vi "一体站流程质控自动启动.vi"(6 "CODMn量程切换":enum32{"H", "L", "AUTO"}(ring)=enum."AUTO", 8 "总磷量程切换":enum32{"H", "L", "AUTO"}(ring)=enum."AUTO", 9 "总氮量程切换":enum32{"H", "L", "AUTO"}(ring)=enum."AUTO", 10 "氨氮量程切换":enum32{"H", "L", "AUTO"}(ring)=enum."AUTO", 11 "参数":T1={"是否启用仪器"=FALSE, "CODMn"={"启动测量模式"={"测量模式"=enum."水样测量"}, "确定按钮"=TRUE}, "启动模块"={"氨氮"=FALSE, "总磷"=FALSE, "总氮"=FALSE, "CODMn"=FALSE, "CODCr"=FALSE}, "常规启动"=FALSE, "直接启动"=FALSE}) -> ()   [LabVIEW 2016, in "质控单元.lvlib"]
panel:
  out "枚举 2":enum16{"初始化", "采配水启动", "等待", "配水", "排水", "结束"}(ring)
  out "枚举":enum16{"初始化", "采配水启动", "等待", "配水", "排水", "结束"}(ring)
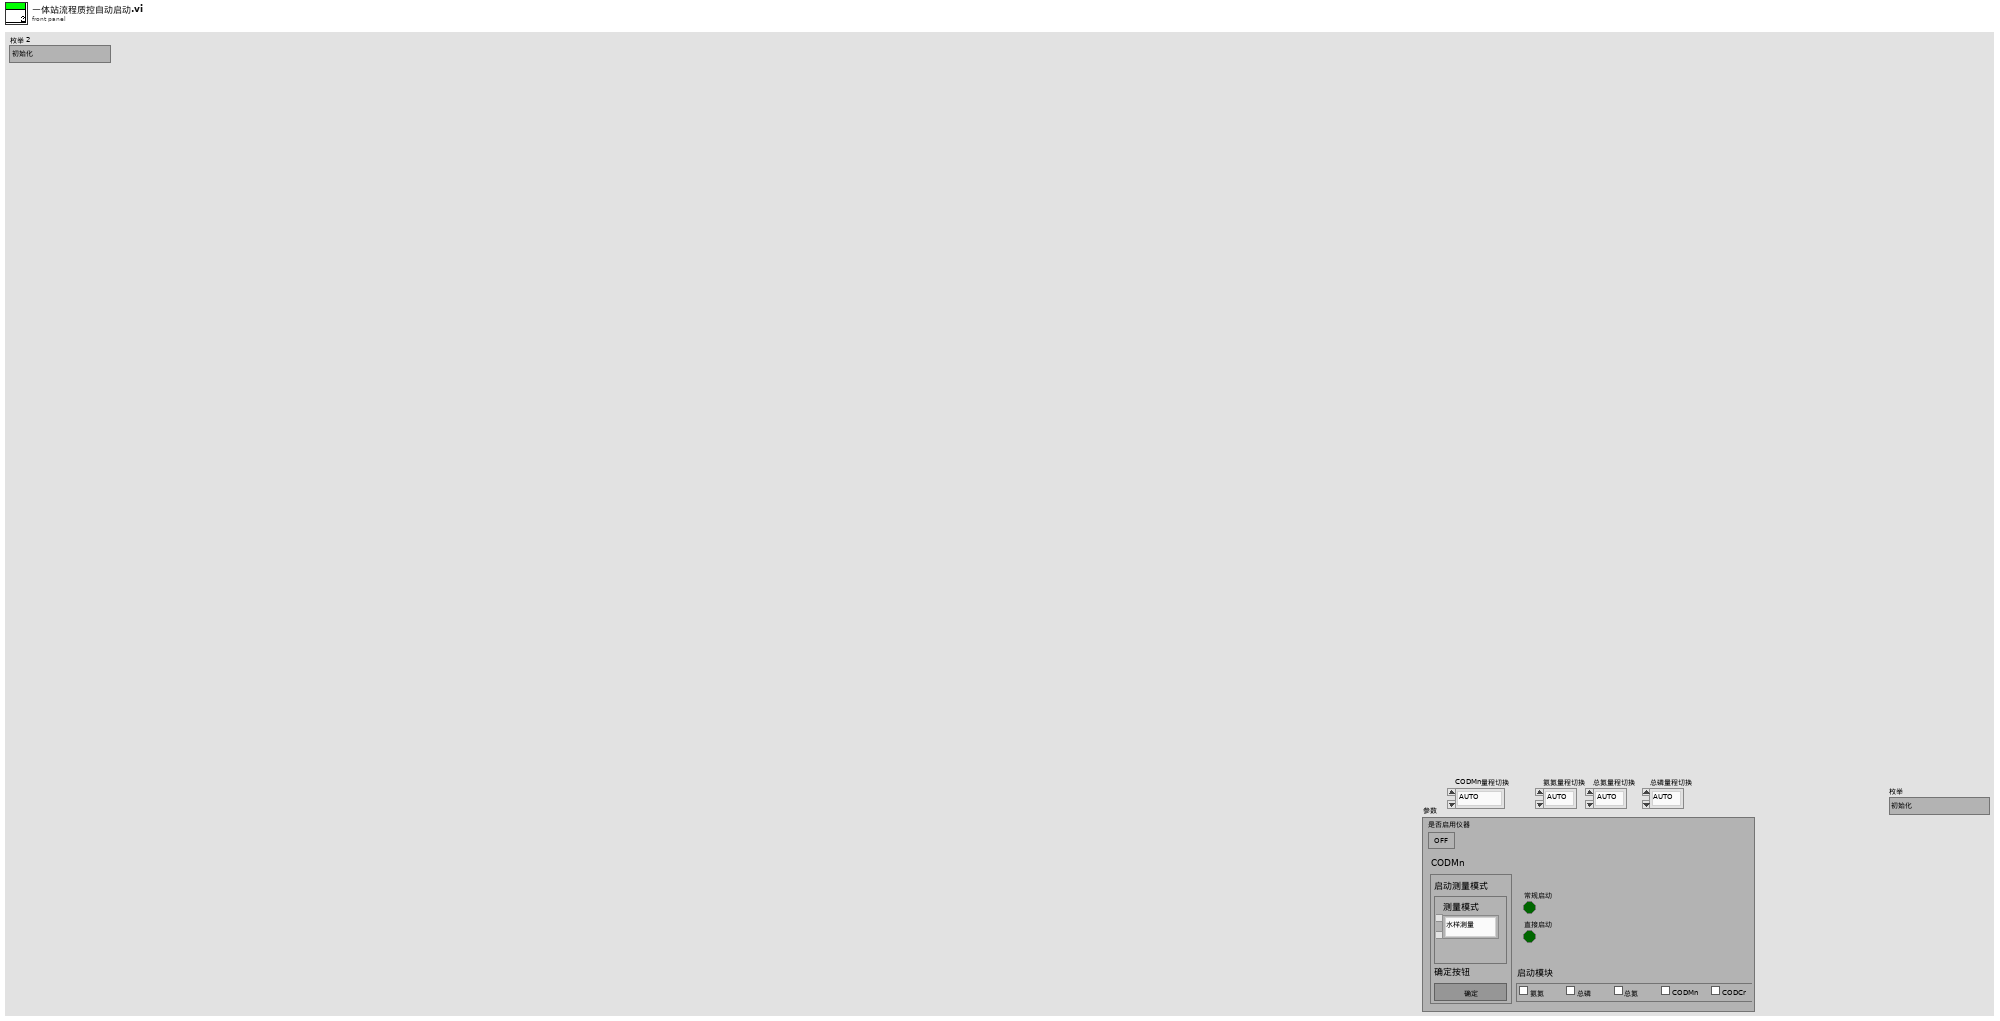
[diagram p1: front panel]
types:
  T1 = cluster{"是否启用仪器":bool, "CODMn":cluster{"启动测量模式":cluster{"测量模式":enum16{"水样测量", "标样核查", "加标回收", "平行样", "校零", "校标"}}, "确定按钮":bool}, "启动模块":cluster{"氨氮":bool, "总磷":bool, "总氮":bool, "CODMn":bool, "CODCr":bool}, "常规启动":bool, "直接启动":bool}
  T2 = cluster{"命令":string, cluster{"starting address":u16, "holding register value":u16}}
  T3 = cluster{"R0":i16, "R1":i16, "R2":i16, "R3":i16, "R4":i16, "R5":i16, "R6":i16, "R7":i16, "R8":i16, "R9":i16, "R10":i16, "R11":i16, "R12":i16, "R13":i16, "R14":i16, "R15":i16, "R16":i16, "R17":i16, "R18":i16, "R19":i16, "R20":i16, "R21":i16, "R22":i16, "R23":i16, "R24":i16, "R25":i16, "R26":i16, "R27":i16, "R28":i16, "R29":i16, "R30":i16, "R31":i16, "R32":i16, "R33":i16, "R34":i16, "R35":i16, "R36":i16, "R37":i16, "R38":i16, "R39":i16, "R40":i16, "R41":i16, "R42":i16, "R43":i16, "R44":i16, "R45":i16, "R46":i16, "R47":i16, "R48":i16, "R49":i16, "R50":i16, "R51":i16, "R52":i16, "R53":i16, "R54":i16, "R55":i16, "R56":i16}
  T4 = enum32{"Bad", "Idle", "Run top level", "Running"}
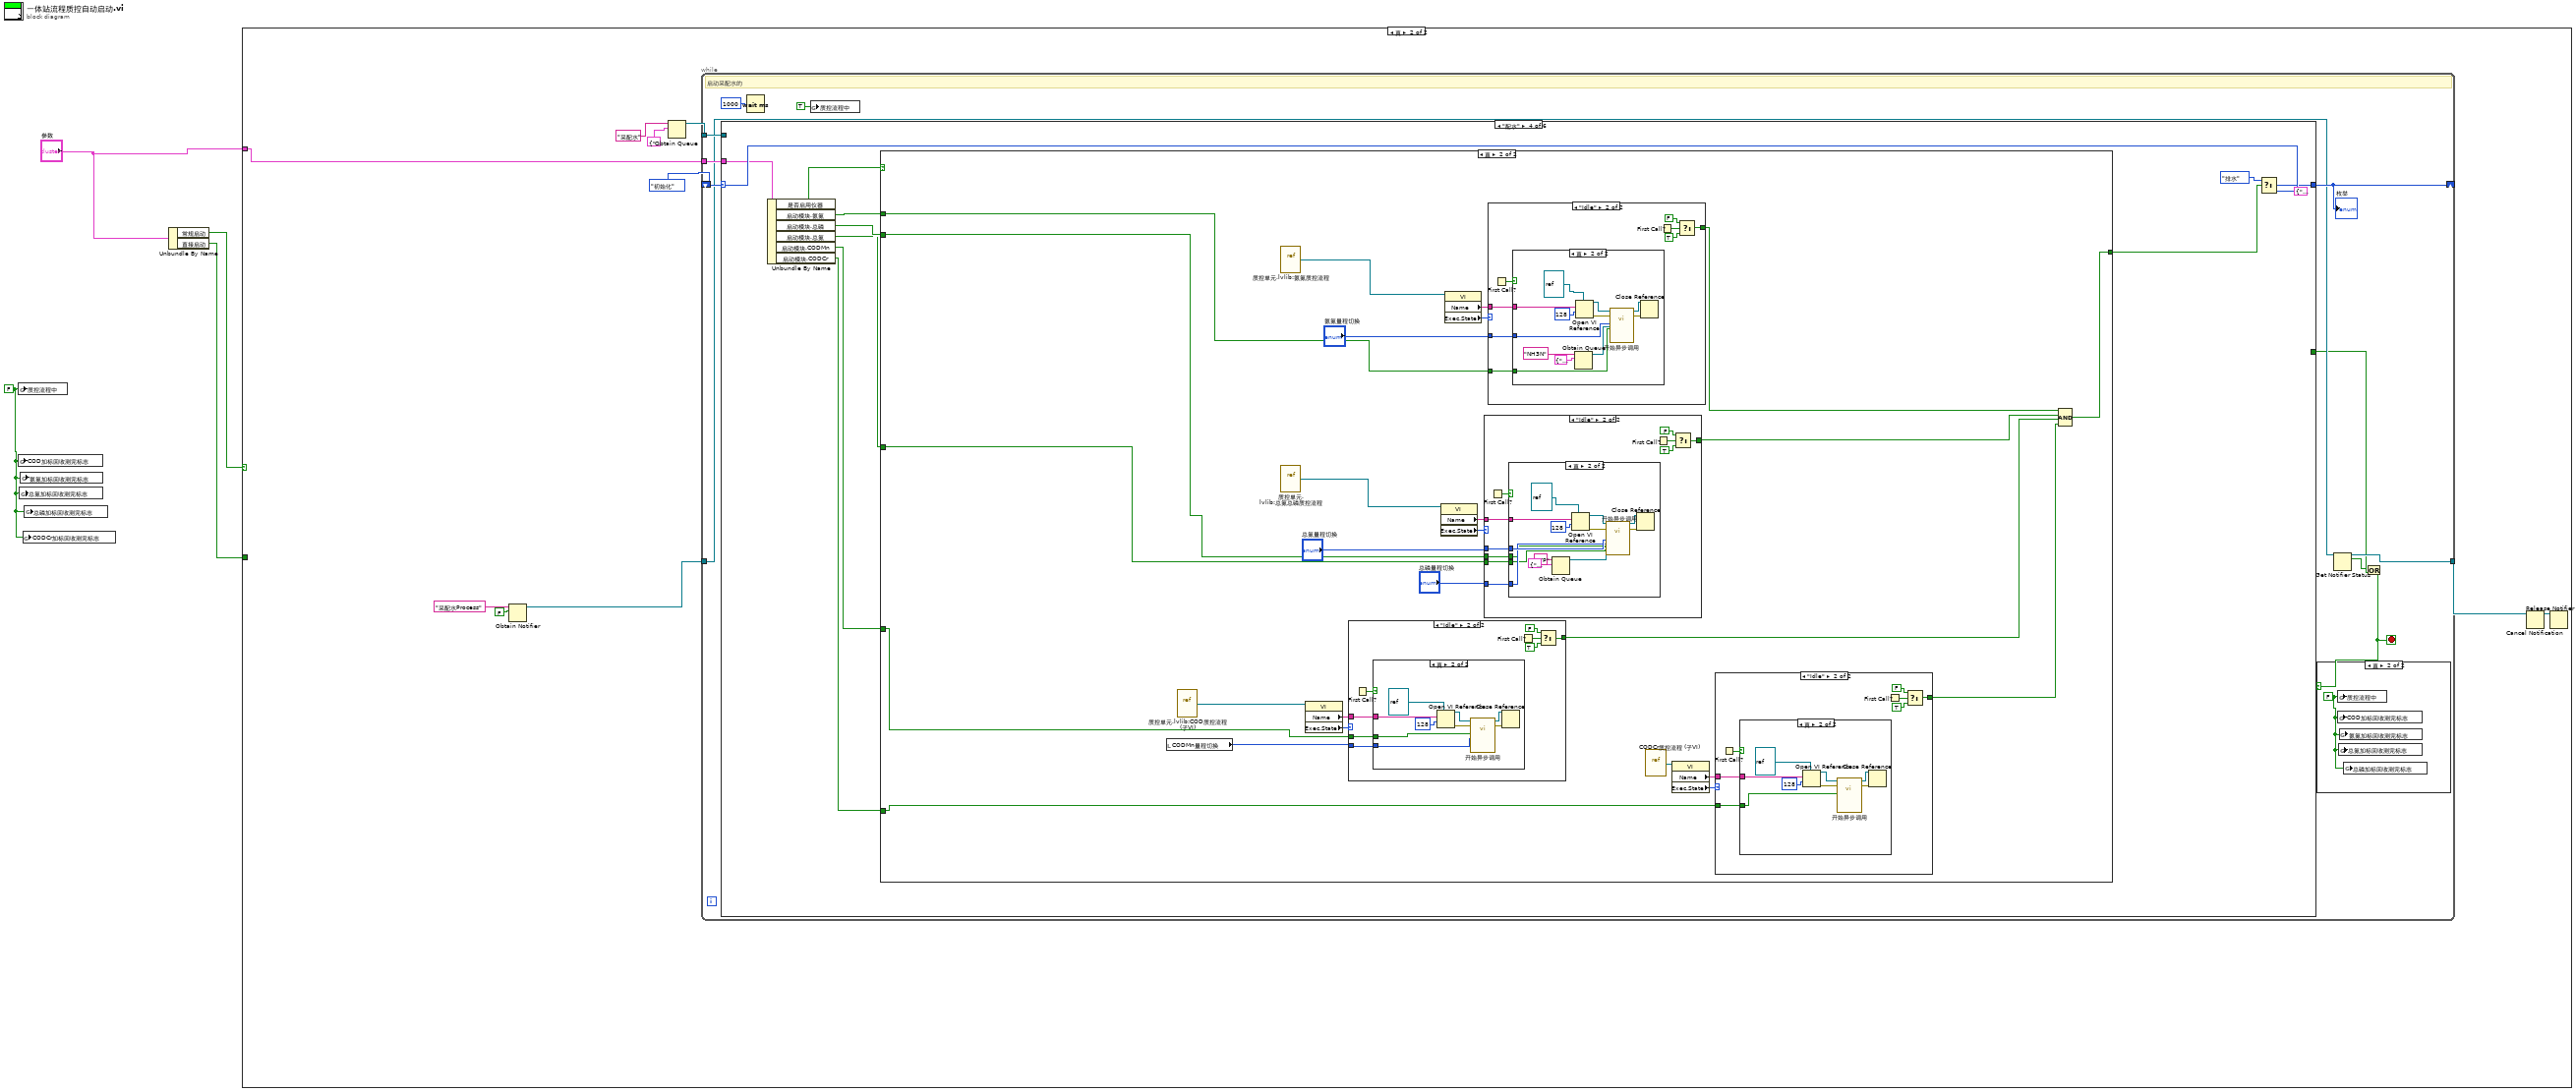
[diagram p0: block diagram]
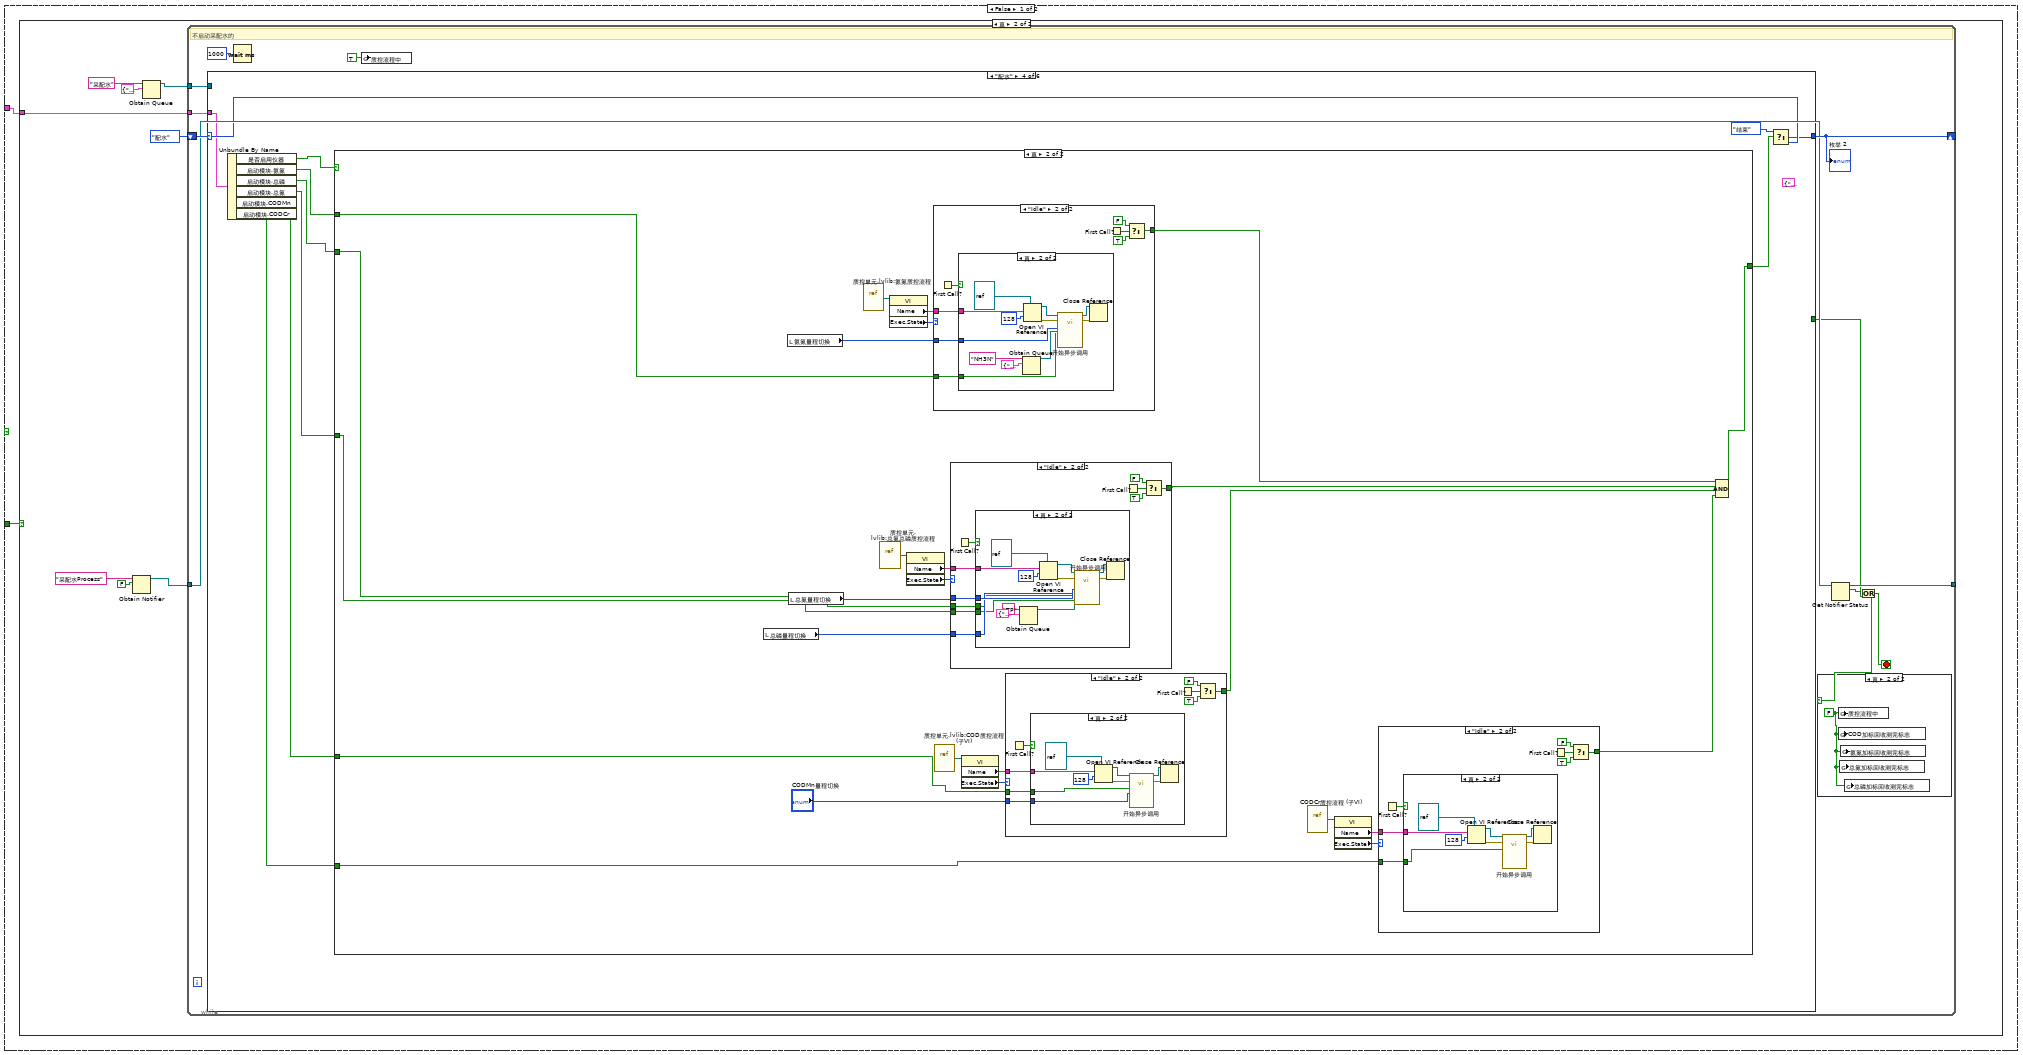
[diagram p2: hidden frame]
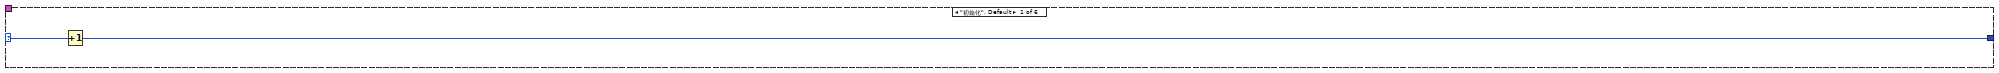
[diagram p5: hidden frame]
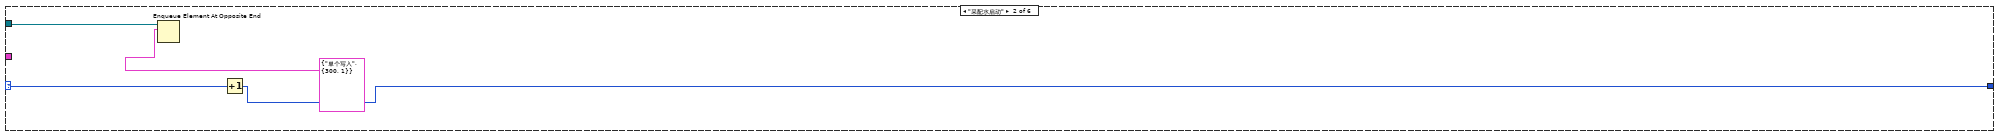
[diagram p6: hidden frame]
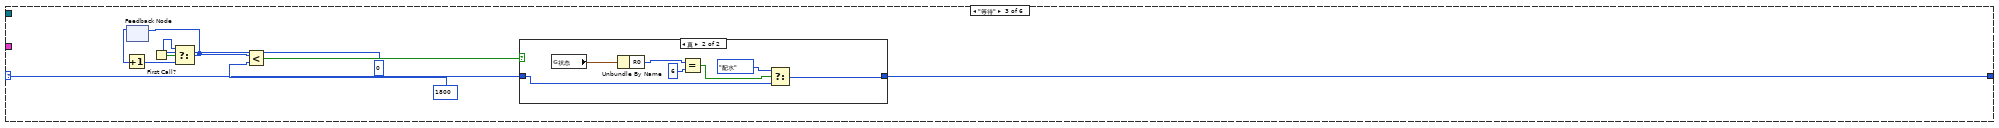
[diagram p7: hidden frame]
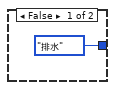
[diagram p8: hidden frame]
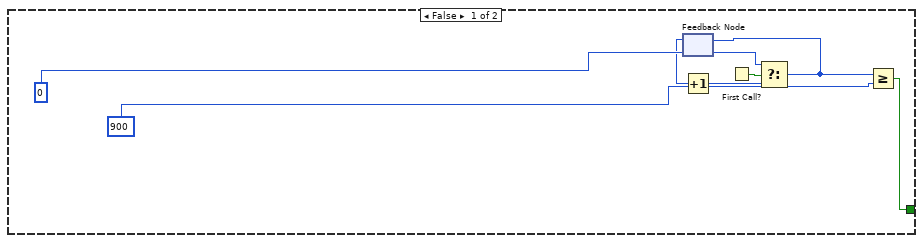
[diagram p9: hidden frame]
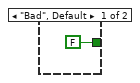
[diagram p10: hidden frame]
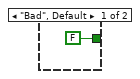
[diagram p12: hidden frame]
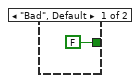
[diagram p14: hidden frame]
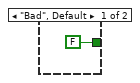
[diagram p16: hidden frame]
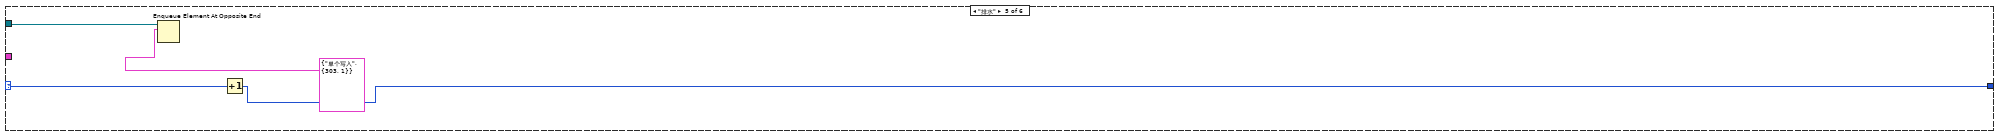
[diagram p18: hidden frame]
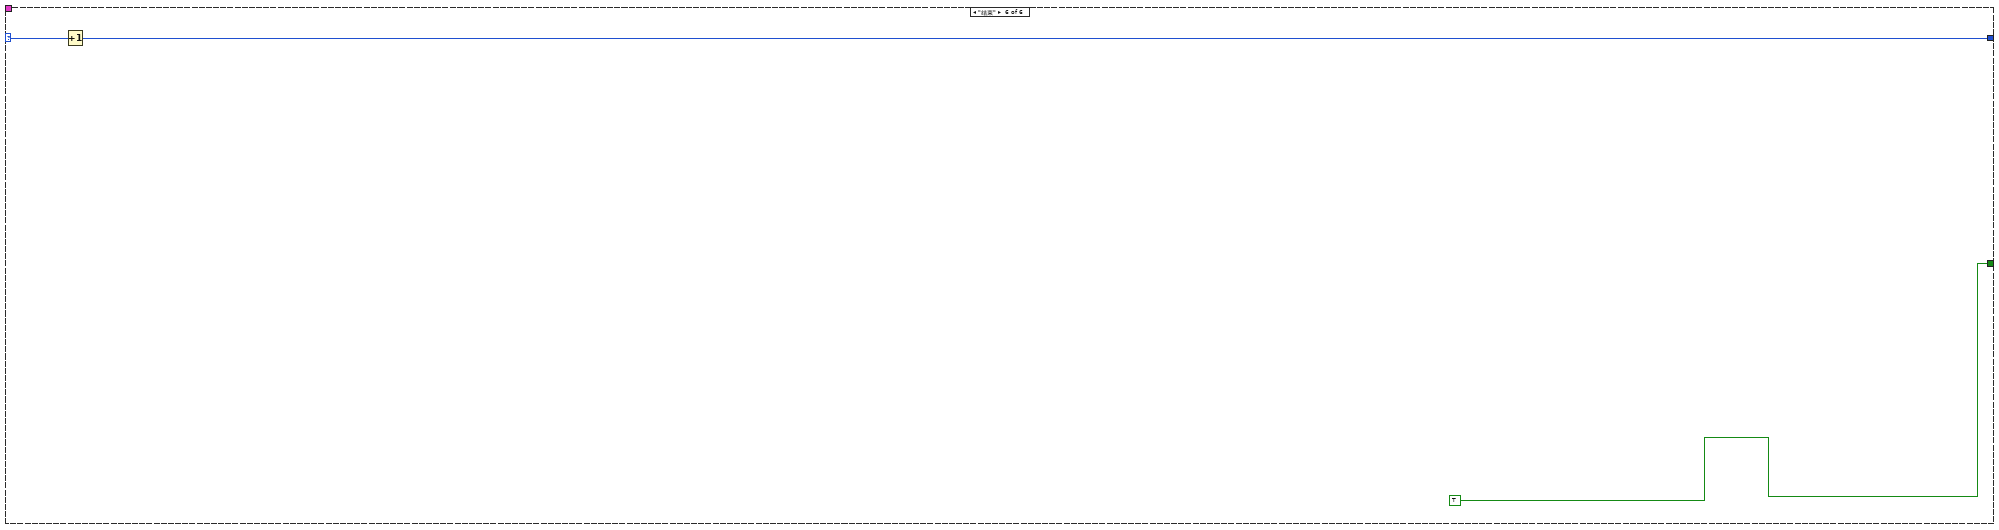
[diagram p19: hidden frame]
diagram:
  w1 = FALSE ("质控流程中")
  n1 = global write "质控测完标志全局 1.vi" "质控流程中"(w1) -> ()
  n2 = global write "质控测完标志全局 1.vi" "COD加标回收测完标志"(w1) -> ()
  n3 = global write "质控测完标志全局 1.vi" "总氮加标回收测完标志"(w1) -> ()
  n4 = global write "质控测完标志全局 1.vi" "氨氮加标回收测完标志"(w1) -> ()
  n5 = global write "质控测完标志全局 1.vi" "CODCr加标回收测完标志"(w1) -> ()
  n6 = global write "质控测完标志全局 1.vi" "总磷加标回收测完标志"(w1) -> ()
  n7 = Unbundle By Name("参数") -> ("常规启动"=w3:bool, "直接启动"=w2:bool)
  n8 = case shown="真" w3 {
    tunnel: "参数" -> [w5 w181]
    tunnel: w2 -> [w6 _]
    frame False {
      n9 = case shown="真" w6 {
        tunnel: w5 -> [_ w13]
        frame False {
        }
        frame True {
          n10 = Obtain Notifier(name (unnamed)="采配水Process" ("名称（未命名）"), notification data type=FALSE) -> (notifier out=w7:refnum<notifier>)  [unwired: 2 in, 2 out]
          n11 = Obtain Queue(name (unnamed)="采配水" ("名称（未命名）"), element data type=cluster{"命令":string, "数据":variant} {"命令"="", "数据"=variant}) -> (queue out=w10:refnum<queue>)  [unwired: 3 in, 2 out]
          n12 = while {
            tunnel: w10 -> [w25]
            shift-right: [w23] -> _
            shift-left: enum16{"初始化", "采配水启动", "等待", "配水", "排水", "结束"}."配水" ("枚举") -> [w24]
            tunnel: w13 -> [w21]
            tunnel: w7 -> [w20]
            tunnel: [w19] -> _
            stop <- w16 stop-if-true
            # "不启动采配水的"
            n13 = case shown="\"配水\"" w24 {
              selector: w24 -> [w28 w30 w39 w59 w175 w180]
              tunnel: w25 -> [_ w31 _ _ w176 _]
              tunnel: [w27 w29 w38 w58 w174 w179] -> w23
              tunnel: [_ _ _ _ _ TRUE] -> w18
              tunnel: w21 -> [_ _ _ w55 _ _]
              frame "初始化", Default {
                n14 = Increment(x=w28) -> (x+1=w27:enum16{"初始化", "采配水启动", "等待", "配水", "排水", "结束"})
              }
              frame "采配水启动" {
                n15 = Enqueue Element At Opposite End(queue=w31, element=T2 {"命令"="单个写入", {"starting address"=300, "holding register value"=1}} ("元素")) -> ()  [unwired: 2 in, 3 out]
                n16 = Increment(x=w30) -> (x+1=w29:enum16{"初始化", "采配水启动", "等待", "配水", "排水", "结束"})
              }
              frame "等待" {
                n17 = feedback #1() -> (w35:i32)  [unwired: 1 in]
                n18 = Increment(x=w35) -> (x+1=w34:i32)
                n19 = First Call?() -> (First Call?: T/F=w36:bool)
                n20 = Select(t=0, s=w36, f=w34) -> (s? t:f=w33:i32)
                n21 = feedback-in #1(w33) -> ()
                n22 = Less?(x=w33, y=1800) -> (x < y?=w40:bool)
                n23 = case shown="真" w40 {
                  tunnel: w39 -> [_ w45]
                  tunnel: [enum16{"初始化", "采配水启动", "等待", "配水", "排水", "结束"}."排水" ("枚举") w44] -> w38
                  frame False {
                  }
                  frame True {
                    n24 = global read "与采配水交互全局.vi" "状态"() -> (w43:T3)
                    n25 = Unbundle By Name(w43) -> ("R0"=w49:i16)
                    n26 = Equal?(x=w49, y=i16 6) -> (x = y?=w47:bool)
                    n27 = Select(t=enum16{"初始化", "采配水启动", "等待", "配水", "排水", "结束"}."配水" ("枚举"), s=w47, f=w45) -> (s? t:f=w44:enum16{"初始化", "采配水启动", "等待", "配水", "排水", "结束"})
                  }
                }
              }
              frame "配水" {
                (unwired) cluster{"命令":string, "data":variant} {"命令"="启动", "data"=variant(cluster{"站号":u16, "控制命令输出":u16[]} {"站号"=1, "控制命令输出"=[256, 0]})} ("元素")
                n28 = Unbundle By Name(w55) -> ("是否启用仪器"=w57:bool, "启动模块.氨氮"=w53:bool, "启动模块.总磷"=w54:bool, "启动模块.总氮"=w51:bool, "启动模块.CODMn"=w52:bool, "启动模块.CODCr"=w50:bool)
                n29 = case shown="真" w57 {
                  tunnel: [w61 w93] -> w56
                  tunnel: w54 -> [_ w81]
                  tunnel: w53 -> [_ w89]
                  tunnel: w52 -> [_ w72]
                  tunnel: w51 -> [_ w80]
                  tunnel: w50 -> [_ w69]
                  frame False {
                    n30 = feedback #2() -> (w65:i32)  [unwired: 1 in]
                    n31 = Increment(x=w65) -> (x+1=w64:i32)
                    n32 = First Call?() -> (First Call?: T/F=w66:bool)
                    n33 = Select(t=0, s=w66, f=w64) -> (s? t:f=w62:i32)
                    n34 = feedback-in #2(w62) -> ()
                    n35 = Greater Or Equal?(x=w62, y=900) -> (x >= y?=w61:bool)
                  }
                  frame True {
                    n36 = local read "总磷量程切换"() -> (w82:enum32{"H", "L", "AUTO"})
                    n37 = local read "氨氮量程切换"() -> (w87:enum32{"H", "L", "AUTO"})
                    n38 = local read "总氮量程切换"() -> (w83:enum32{"H", "L", "AUTO"})
                    n39 = vi-ref "质控单元.lvlib:氨氮质控流程.vi"() -> (w91:refnum<vi>)
                    n40 = vi-ref "质控单元.lvlib:总氮总磷质控流程.vi"() -> (w85:refnum<vi>)
                    n41 = property class="VI"(reference=w91) -> ("Name"=w92:string, "Exec.State"=w90:T4)  [unwired: 1 in, 2 out]
                    n42 = property class="VI"(reference=w85) -> ("Name"=w84:string, "Exec.State"=w86:T4)  [unwired: 1 in, 2 out]
                    n43 = case shown="\"Idle\"" w90 {
                      tunnel: w92 -> [_ w161]
                      tunnel: w89 -> [_ w160]
                      tunnel: [FALSE w155] -> w88
                      tunnel: w87 -> [_ w154]
                      frame "Bad", Default {
                      }
                      frame "Idle" {
                        n44 = First Call?() -> (First Call?: T/F=w159:bool)
                        n45 = case shown="真" w159 {
                          tunnel: w161 -> [_ w172]
                          tunnel: w160 -> [_ w163]
                          tunnel: w154 -> [_ w162]
                          frame False {
                          }
                          frame True {
                            n46 = Obtain Queue(name (unnamed)="NH3N" ("名称（未命名）"), element data type=cluster{"命令":string, "data":variant} {"命令"="", "data"=variant}) -> (queue out=w164:refnum<queue>)  [unwired: 3 in, 2 out]
                            n47 = Open VI Reference(type specifier VI Refnum (for type only)=refnum<vi> refnum ("类型说明符VI引用句柄（仅用于类型）"), vi path=w172, options=128 ("选项")) -> (vi reference=w173:refnum<vi>, error out=w169:errorcluster)  [unwired: 3 in]
                            n48 = call-by-ref "开始异步调用"(reference=w173, error in=w169, "队列输入NH3"=w164, "氨氮"=w163, "氨氮量程切换"=w162) -> (reference out=w171:refnum<vi>, error out=w170:errorcluster)  [unwired: 7 in, 2 out]
                            n49 = Close Reference(reference=w171, error in (no error)=w170) -> ()  [unwired: 1 out]
                          }
                        }
                        n50 = First Call?() -> (First Call?: T/F=w158:bool)
                        n51 = Select(t=FALSE, s=w158, f=TRUE) -> (s? t:f=w155:bool)
                      }
                    }
                    n52 = vi-ref "质控单元.lvlib:COD质控流程 (子VI).vi"() -> (w77:refnum<vi>)
                    n53 = case shown="\"Idle\"" w86 {
                      tunnel: w84 -> [_ w138]
                      tunnel: w82 -> [_ w137]
                      tunnel: [FALSE w132] -> w79
                      tunnel: w83 -> [_ w131]
                      tunnel: w81 -> [_ w130]
                      tunnel: w80 -> [_ w129]
                      frame "Bad", Default {
                      }
                      frame "Idle" {
                        n54 = First Call?() -> (First Call?: T/F=w136:bool)
                        n55 = case shown="真" w136 {
                          tunnel: w138 -> [_ w152]
                          tunnel: w137 -> [_ w141]
                          tunnel: w131 -> [_ w142]
                          tunnel: w130 -> [_ w140]
                          tunnel: w129 -> [_ w139]
                          frame False {
                          }
                          frame True {
                            n56 = Obtain Queue(name (unnamed)="TP" ("名称（未命名）"), element data type=cluster{"命令":string, "data":variant} {"命令"="", "data"=variant}) -> (queue out=w143:refnum<queue>)  [unwired: 3 in, 2 out]
                            n57 = Open VI Reference(type specifier VI Refnum (for type only)=refnum<vi> refnum ("类型说明符VI引用句柄（仅用于类型）"), vi path=w152, options=128 ("选项")) -> (vi reference=w144:refnum<vi>, error out=w149:errorcluster)  [unwired: 3 in]
                            n58 = call-by-ref "开始异步调用"(reference=w144, error in=w149, "队列输入TP"=w143, "总氮量程切换"=w142, "总磷量程切换"=w141, "总磷"=w140, "总氮"=w139) -> (reference out=w151:refnum<vi>, error out=w150:errorcluster)  [unwired: 8 in, 3 out]
                            n59 = Close Reference(reference=w151, error in (no error)=w150) -> ()  [unwired: 1 out]
                          }
                        }
                        n60 = First Call?() -> (First Call?: T/F=w135:bool)
                        n61 = Select(t=FALSE, s=w135, f=TRUE) -> (s? t:f=w132:bool)
                      }
                    }
                    n62 = property class="VI"(reference=w77) -> ("Name"=w78:string, "Exec.State"=w76:T4)  [unwired: 1 in, 2 out]
                    n63 = case shown="\"Idle\"" w76 {
                      tunnel: w78 -> [_ w118]
                      tunnel: [FALSE w113] -> w70
                      tunnel: "CODMn量程切换" -> [_ w112]
                      tunnel: w72 -> [_ w111]
                      frame "Bad", Default {
                      }
                      frame "Idle" {
                        n64 = First Call?() -> (First Call?: T/F=w117:bool)
                        n65 = case shown="真" w117 {
                          tunnel: w118 -> [_ w126]
                          tunnel: w112 -> [_ w119]
                          tunnel: w111 -> [_ w120]
                          frame False {
                          }
                          frame True {
                            n66 = Open VI Reference(type specifier VI Refnum (for type only)=refnum<vi> refnum ("类型说明符VI引用句柄（仅用于类型）"), vi path=w126, options=128 ("选项")) -> (vi reference=w127:refnum<vi>, error out=w123:errorcluster)  [unwired: 3 in]
                            n67 = call-by-ref "开始异步调用"(reference=w127, error in=w123, "CODMn量程切换"=w119, "COD"=w120) -> (reference out=w125:refnum<vi>, error out=w124:errorcluster)  [unwired: 8 in, 2 out]
                            n68 = Close Reference(reference=w125, error in (no error)=w124) -> ()  [unwired: 1 out]
                          }
                        }
                        n69 = First Call?() -> (First Call?: T/F=w116:bool)
                        n70 = Select(t=FALSE, s=w116, f=TRUE) -> (s? t:f=w113:bool)
                      }
                    }
                    n71 = vi-ref "CODCr质控流程 (子VI).vi"() -> (w74:refnum<vi>)
                    n72 = property class="VI"(reference=w74) -> ("Name"=w75:string, "Exec.State"=w73:T4)  [unwired: 1 in, 2 out]
                    n73 = case shown="\"Idle\"" w73 {
                      tunnel: w75 -> [_ w101]
                      tunnel: [FALSE w96] -> w68
                      tunnel: w69 -> [_ w95]
                      frame "Bad", Default {
                      }
                      frame "Idle" {
                        n74 = First Call?() -> (First Call?: T/F=w100:bool)
                        n75 = case shown="真" w100 {
                          tunnel: w101 -> [_ w108]
                          tunnel: w95 -> [_ w102]
                          frame False {
                          }
                          frame True {
                            n76 = Open VI Reference(type specifier VI Refnum (for type only)=refnum<vi> refnum ("类型说明符VI引用句柄（仅用于类型）"), vi path=w108, options=128 ("选项")) -> (vi reference=w109:refnum<vi>, error out=w105:errorcluster)  [unwired: 3 in]
                            n77 = call-by-ref "开始异步调用"(reference=w109, error in=w105, "CODCr"=w102) -> (reference out=w107:refnum<vi>, error out=w106:errorcluster)  [unwired: 9 in, 2 out]
                            n78 = Close Reference(reference=w107, error in (no error)=w106) -> ()  [unwired: 1 out]
                          }
                        }
                        n79 = First Call?() -> (First Call?: T/F=w99:bool)
                        n80 = Select(t=FALSE, s=w99, f=TRUE) -> (s? t:f=w96:bool)
                      }
                    }
                    n81 = Compound Arithmetic op=AND ("复合运算")(w88, w79, w70, w68) -> (w93:bool)
                  }
                }
                n82 = Select(t=enum16{"初始化", "采配水启动", "等待", "配水", "排水", "结束"}."结束" ("枚举"), s=w56, f=w59) -> (s? t:f=w58:enum16{"初始化", "采配水启动", "等待", "配水", "排水", "结束"})
              }
              frame "排水" {
                n83 = Enqueue Element At Opposite End(queue=w176, element=T2 {"命令"="单个写入", {"starting address"=303, "holding register value"=1}} ("元素")) -> ()  [unwired: 2 in, 3 out]
                n84 = Increment(x=w175) -> (x+1=w174:enum16{"初始化", "采配水启动", "等待", "配水", "排水", "结束"})
              }
              frame "结束" {
                n85 = Increment(x=w180) -> (x+1=w179:enum16{"初始化", "采配水启动", "等待", "配水", "排水", "结束"})
              }
            }
            "枚举 2" <- w23
            n86 = Wait (ms)(milliseconds to wait=u32 1000 ("等待时间（毫秒）")) -> ()  [unwired: 1 out]
            n87 = global write "质控测完标志全局 1.vi" "质控流程中"(TRUE ("质控流程中")) -> ()
            n88 = Get Notifier Status(notifier=w20) -> (notifier out=w19:refnum<notifier>, current notification=w17:bool)  [unwired: 1 in, 3 out]
            n89 = Or(x=w17, y=w18) -> (x .or. y?=w16:bool)
            n90 = case shown="真" w16 {
              frame False {
              }
              frame True {
                w26 = FALSE ("质控流程中")
                n91 = global write "质控测完标志全局 1.vi" "质控流程中"(w26) -> ()
                n92 = global write "质控测完标志全局 1.vi" "COD加标回收测完标志"(w26) -> ()
                n93 = global write "质控测完标志全局 1.vi" "总氮加标回收测完标志"(w26) -> ()
                n94 = global write "质控测完标志全局 1.vi" "氨氮加标回收测完标志"(w26) -> ()
                n95 = global write "质控测完标志全局 1.vi" "总磷加标回收测完标志"(w26) -> ()
              }
            }
          }
        }
      }
    }
    frame True {
      n96 = Obtain Notifier(name (unnamed)="采配水Process" ("名称（未命名）"), notification data type=FALSE) -> (notifier out=w184:refnum<notifier>)  [unwired: 2 in, 2 out]
      n97 = Obtain Queue(name (unnamed)="采配水" ("名称（未命名）"), element data type=cluster{"命令":string, "数据":variant} {"命令"="", "数据"=variant}) -> (queue out=w188:refnum<queue>)  [unwired: 3 in, 2 out]
      n98 = while {
        tunnel: w188 -> [w201]
        shift-right: [w199] -> _
        shift-left: enum16{"初始化", "采配水启动", "等待", "配水", "排水", "结束"}."初始化" ("枚举") -> [w200]
        tunnel: w181 -> [w197]
        tunnel: w184 -> [w196]
        tunnel: [w195] -> w183
        stop <- w192 stop-if-true
        # "启动采配水的"
        n99 = case shown="\"配水\"" w200 {
          selector: w200 -> [w204 w208 w217 w237 w353 w358]
          tunnel: w201 -> [_ w209 _ _ w354 _]
          tunnel: [w203 w207 w216 w236 w352 w357] -> w199
          tunnel: [_ _ _ _ _ TRUE] -> w194
          tunnel: w197 -> [_ _ _ w233 _ _]
          frame "初始化", Default {
            n100 = Increment(x=w204) -> (x+1=w203:enum16{"初始化", "采配水启动", "等待", "配水", "排水", "结束"})
          }
          frame "采配水启动" {
            n101 = Enqueue Element At Opposite End(queue=w209, element=T2 {"命令"="单个写入", {"starting address"=300, "holding register value"=1}} ("元素")) -> (queue out=w205:refnum<queue>)  [unwired: 2 in, 2 out]
            n102 = Increment(x=w208) -> (x+1=w207:enum16{"初始化", "采配水启动", "等待", "配水", "排水", "结束"})
            n103 = Enqueue Element At Opposite End(queue=w205, element=T2 {"命令"="单个写入", {"starting address"=303, "holding register value"=1}} ("元素")) -> ()  [unwired: 2 in, 3 out]
          }
          frame "等待" {
            n104 = feedback #3() -> (w213:i32)  [unwired: 1 in]
            n105 = Increment(x=w213) -> (x+1=w212:i32)
            n106 = First Call?() -> (First Call?: T/F=w214:bool)
            n107 = Select(t=0, s=w214, f=w212) -> (s? t:f=w211:i32)
            n108 = feedback-in #3(w211) -> ()
            n109 = Less?(x=w211, y=1800) -> (x < y?=w218:bool)
            n110 = case shown="真" w218 {
              tunnel: w217 -> [_ w223]
              tunnel: [enum16{"初始化", "采配水启动", "等待", "配水", "排水", "结束"}."排水" ("枚举") w222] -> w216
              frame False {
              }
              frame True {
                n111 = global read "与采配水交互全局.vi" "状态"() -> (w221:T3)
                n112 = Unbundle By Name(w221) -> ("R0"=w227:i16)
                n113 = Equal?(x=w227, y=i16 6) -> (x = y?=w225:bool)
                n114 = Select(t=enum16{"初始化", "采配水启动", "等待", "配水", "排水", "结束"}."配水" ("枚举"), s=w225, f=w223) -> (s? t:f=w222:enum16{"初始化", "采配水启动", "等待", "配水", "排水", "结束"})
              }
            }
          }
          frame "配水" {
            (unwired) cluster{"命令":string, "data":variant} {"命令"="启动", "data"=variant(cluster{"站号":u16, "控制命令输出":u16[]} {"站号"=1, "控制命令输出"=[256, 0]})} ("元素")
            n115 = Unbundle By Name(w233) -> ("是否启用仪器"=w235:bool, "启动模块.氨氮"=w231:bool, "启动模块.总磷"=w232:bool, "启动模块.总氮"=w229:bool, "启动模块.CODMn"=w230:bool, "启动模块.CODCr"=w228:bool)
            n116 = case shown="真" w235 {
              tunnel: [w239 w271] -> w234
              tunnel: w232 -> [_ w260]
              tunnel: w231 -> [_ w266]
              tunnel: w230 -> [_ w249]
              tunnel: w229 -> [_ w259]
              tunnel: w228 -> [_ w248]
              frame False {
                n117 = feedback #4() -> (w243:i32)  [unwired: 1 in]
                n118 = Increment(x=w243) -> (x+1=w242:i32)
                n119 = First Call?() -> (First Call?: T/F=w244:bool)
                n120 = Select(t=0, s=w244, f=w242) -> (s? t:f=w240:i32)
                n121 = feedback-in #4(w240) -> ()
                n122 = Greater Or Equal?(x=w240, y=900) -> (x >= y?=w239:bool)
              }
              frame True {
                n123 = local read "CODMn量程切换"() -> (w250:enum32{"H", "L", "AUTO"})
                n124 = vi-ref "质控单元.lvlib:COD质控流程 (子VI).vi"() -> (w255:refnum<vi>)
                n125 = vi-ref "质控单元.lvlib:氨氮质控流程.vi"() -> (w269:refnum<vi>)
                n126 = vi-ref "质控单元.lvlib:总氮总磷质控流程.vi"() -> (w264:refnum<vi>)
                n127 = property class="VI"(reference=w255) -> ("Name"=w256:string, "Exec.State"=w254:T4)  [unwired: 1 in, 2 out]
                n128 = case shown="\"Idle\"" w254 {
                  tunnel: w256 -> [_ w296]
                  tunnel: [FALSE w291] -> w247
                  tunnel: w250 -> [_ w290]
                  tunnel: w249 -> [_ w289]
                  frame "Bad", Default {
                  }
                  frame "Idle" {
                    n129 = First Call?() -> (First Call?: T/F=w295:bool)
                    n130 = case shown="真" w295 {
                      tunnel: w296 -> [_ w304]
                      tunnel: w290 -> [_ w297]
                      tunnel: w289 -> [_ w298]
                      frame False {
                      }
                      frame True {
                        n131 = Open VI Reference(type specifier VI Refnum (for type only)=refnum<vi> refnum ("类型说明符VI引用句柄（仅用于类型）"), vi path=w304, options=128 ("选项")) -> (vi reference=w305:refnum<vi>, error out=w301:errorcluster)  [unwired: 3 in]
                        n132 = call-by-ref "开始异步调用"(reference=w305, error in=w301, "CODMn量程切换"=w297, "COD"=w298) -> (reference out=w303:refnum<vi>, error out=w302:errorcluster)  [unwired: 8 in, 2 out]
                        n133 = Close Reference(reference=w303, error in (no error)=w302) -> ()  [unwired: 1 out]
                      }
                    }
                    n134 = First Call?() -> (First Call?: T/F=w294:bool)
                    n135 = Select(t=FALSE, s=w294, f=TRUE) -> (s? t:f=w291:bool)
                  }
                }
                n136 = property class="VI"(reference=w264) -> ("Name"=w263:string, "Exec.State"=w265:T4)  [unwired: 1 in, 2 out]
                n137 = property class="VI"(reference=w269) -> ("Name"=w270:string, "Exec.State"=w268:T4)  [unwired: 1 in, 2 out]
                n138 = case shown="\"Idle\"" w265 {
                  tunnel: w263 -> [_ w316]
                  tunnel: "总磷量程切换" -> [_ w315]
                  tunnel: [FALSE w310] -> w261
                  tunnel: "总氮量程切换" -> [_ w309]
                  tunnel: w260 -> [_ w308]
                  tunnel: w259 -> [_ w307]
                  frame "Bad", Default {
                  }
                  frame "Idle" {
                    n139 = First Call?() -> (First Call?: T/F=w314:bool)
                    n140 = case shown="真" w314 {
                      tunnel: w316 -> [_ w330]
                      tunnel: w315 -> [_ w320]
                      tunnel: w309 -> [_ w321]
                      tunnel: w308 -> [_ w319]
                      tunnel: w307 -> [_ w318]
                      frame False {
                      }
                      frame True {
                        n141 = Obtain Queue(name (unnamed)="TP" ("名称（未命名）"), element data type=cluster{"命令":string, "data":variant} {"命令"="", "data"=variant}) -> (queue out=w322:refnum<queue>)  [unwired: 3 in, 2 out]
                        n142 = Open VI Reference(type specifier VI Refnum (for type only)=refnum<vi> refnum, vi path=w330, options=128 ("选项")) -> (vi reference=w323:refnum<vi>, error out=w327:errorcluster)  [unwired: 3 in]
                        n143 = call-by-ref "开始异步调用"(reference=w323, error in=w327, "队列输入TP"=w322, "总氮量程切换"=w321, "总磷量程切换"=w320, "总磷"=w319, "总氮"=w318) -> (reference out=w329:refnum<vi>, error out=w328:errorcluster)  [unwired: 8 in, 3 out]
                        n144 = Close Reference(reference=w329, error in (no error)=w328) -> ()  [unwired: 1 out]
                      }
                    }
                    n145 = First Call?() -> (First Call?: T/F=w313:bool)
                    n146 = Select(t=FALSE, s=w313, f=TRUE) -> (s? t:f=w310:bool)
                  }
                }
                n147 = case shown="\"Idle\"" w268 {
                  tunnel: w270 -> [_ w339]
                  tunnel: w266 -> [_ w338]
                  tunnel: [FALSE w333] -> w262
                  tunnel: "氨氮量程切换" -> [_ w332]
                  frame "Bad", Default {
                  }
                  frame "Idle" {
                    n148 = First Call?() -> (First Call?: T/F=w337:bool)
                    n149 = case shown="真" w337 {
                      tunnel: w339 -> [_ w350]
                      tunnel: w338 -> [_ w342]
                      tunnel: w332 -> [_ w341]
                      frame False {
                      }
                      frame True {
                        n150 = Obtain Queue(name (unnamed)="NH3N" ("名称（未命名）"), element data type=cluster{"命令":string, "data":variant} {"命令"="", "data"=variant}) -> (queue out=w343:refnum<queue>)  [unwired: 3 in, 2 out]
                        n151 = Open VI Reference(type specifier VI Refnum (for type only)=refnum<vi> refnum, vi path=w350, options=128 ("选项")) -> (vi reference=w351:refnum<vi>, error out=w347:errorcluster)  [unwired: 3 in]
                        n152 = call-by-ref "开始异步调用"(reference=w351, error in=w347, "队列输入NH3"=w343, "氨氮"=w342, "氨氮量程切换"=w341) -> (reference out=w349:refnum<vi>, error out=w348:errorcluster)  [unwired: 7 in, 2 out]
                        n153 = Close Reference(reference=w349, error in (no error)=w348) -> ()  [unwired: 1 out]
                      }
                    }
                    n154 = First Call?() -> (First Call?: T/F=w336:bool)
                    n155 = Select(t=FALSE, s=w336, f=TRUE) -> (s? t:f=w333:bool)
                  }
                }
                n156 = vi-ref "CODCr质控流程 (子VI).vi"() -> (w252:refnum<vi>)
                n157 = property class="VI"(reference=w252) -> ("Name"=w253:string, "Exec.State"=w251:T4)  [unwired: 1 in, 2 out]
                n158 = case shown="\"Idle\"" w251 {
                  tunnel: w253 -> [_ w279]
                  tunnel: [FALSE w274] -> w246
                  tunnel: w248 -> [_ w273]
                  frame "Bad", Default {
                  }
                  frame "Idle" {
                    n159 = First Call?() -> (First Call?: T/F=w278:bool)
                    n160 = case shown="真" w278 {
                      tunnel: w279 -> [_ w286]
                      tunnel: w273 -> [_ w280]
                      frame False {
                      }
                      frame True {
                        n161 = Open VI Reference(type specifier VI Refnum (for type only)=refnum<vi> refnum ("类型说明符VI引用句柄（仅用于类型）"), vi path=w286, options=128 ("选项")) -> (vi reference=w287:refnum<vi>, error out=w283:errorcluster)  [unwired: 3 in]
                        n162 = call-by-ref "开始异步调用"(reference=w287, error in=w283, "CODCr"=w280) -> (reference out=w285:refnum<vi>, error out=w284:errorcluster)  [unwired: 9 in, 2 out]
                        n163 = Close Reference(reference=w285, error in (no error)=w284) -> ()  [unwired: 1 out]
                      }
                    }
                    n164 = First Call?() -> (First Call?: T/F=w277:bool)
                    n165 = Select(t=FALSE, s=w277, f=TRUE) -> (s? t:f=w274:bool)
                  }
                }
                n166 = Compound Arithmetic op=AND ("复合运算")(w262, w261, w247, w246) -> (w271:bool)
              }
            }
            n167 = Select(t=enum16{"初始化", "采配水启动", "等待", "配水", "排水", "结束"}."排水" ("枚举"), s=w234, f=w237) -> (s? t:f=w236:enum16{"初始化", "采配水启动", "等待", "配水", "排水", "结束"})
          }
          frame "排水" {
            n168 = Enqueue Element At Opposite End(queue=w354, element=T2 {"命令"="单个写入", {"starting address"=303, "holding register value"=1}} ("元素")) -> ()  [unwired: 2 in, 3 out]
            n169 = Increment(x=w353) -> (x+1=w352:enum16{"初始化", "采配水启动", "等待", "配水", "排水", "结束"})
          }
          frame "结束" {
            n170 = Increment(x=w358) -> (x+1=w357:enum16{"初始化", "采配水启动", "等待", "配水", "排水", "结束"})
          }
        }
        "枚举" <- w199
        n171 = Wait (ms)(milliseconds to wait=u32 1000 ("等待时间（毫秒）")) -> ()  [unwired: 1 out]
        n172 = global write "质控测完标志全局 1.vi" "质控流程中"(TRUE ("质控流程中")) -> ()
        n173 = Get Notifier Status(notifier=w196) -> (notifier out=w195:refnum<notifier>, current notification=w193:bool)  [unwired: 1 in, 3 out]
        n174 = Or(x=w193, y=w194) -> (x .or. y?=w192:bool)
        n175 = case shown="真" w192 {
          frame False {
          }
          frame True {
            w202 = FALSE ("质控流程中")
            n176 = global write "质控测完标志全局 1.vi" "质控流程中"(w202) -> ()
            n177 = global write "质控测完标志全局 1.vi" "COD加标回收测完标志"(w202) -> ()
            n178 = global write "质控测完标志全局 1.vi" "总氮加标回收测完标志"(w202) -> ()
            n179 = global write "质控测完标志全局 1.vi" "氨氮加标回收测完标志"(w202) -> ()
            n180 = global write "质控测完标志全局 1.vi" "总磷加标回收测完标志"(w202) -> ()
          }
        }
      }
      n181 = Cancel Notification(0:w183) -> (8:w182:refnum<notifier>)  [unwired: 1 in, 2 out]
      n182 = Release Notifier(notifier=w182) -> ()  [unwired: 2 in, 3 out]
    }
  }
